vi "Phasor Get Min, Med & Max Decay Indices.vi"(8 "Period":dbl, 9 "Max X":dbl, 10 "Min X":dbl, 11 "X Array":dbl[](array[numeric])) -> (1 "Max X idx":dbl, 2 "Med X idx":dbl, 3 "Min X idx":dbl)   [LabVIEW 2021, in "Phasor.lvlib"]
uses:
  Phasor.lvlib
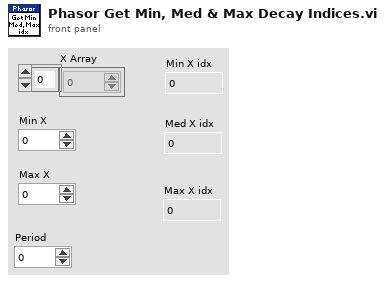
[diagram p1: front panel]
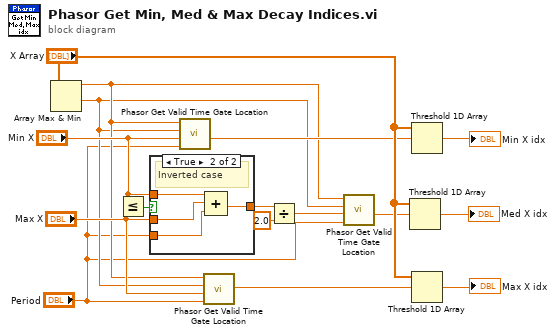
[diagram p0: block diagram]
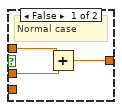
[diagram p2: hidden frame]
diagram:
  n1 = Array Max & Min(array="X Array") -> (max value=w4:dbl, min value=w3:dbl)  [unwired: 2 out]
  n2 = Less Or Equal?(x="Min X", y="Max X") -> (x <= y?=w12:bool)
  n3 = case shown="True" w12 {
    tunnel: "Min X" -> [w19 w23]
    tunnel: "Max X" -> [w18 w22]
    tunnel: "Period" -> [_ w20]
    tunnel: [w17 w21] -> w10
    frame False {
      # "Normal case"
      n4 = Add(x=w19, y=w18) -> (x+y=w17:dbl)
    }
    frame True {
      # "Inverted case"
      n5 = Compound Arithmetic op=ADD(w23, w22, w20) -> (w21:dbl)
    }
  }
  n6 = call "Phasor Get Valid Time Gate Location.vi"("Period"="Period", "X"="Min X", "Min X"=w3, "Max X"=w4) -> ("X in [Min X, Max X]"=w6:dbl)  [unwired: 7 in]
  n7 = call "Phasor Get Valid Time Gate Location.vi"("Period"="Period", "X"="Max X", "Min X"=w3, "Max X"=w4) -> ("X in [Min X, Max X]"=w9:dbl)  [unwired: 7 in]
  n8 = Divide(x=w10, y=2.0) -> (x/y=w5:dbl)
  n9 = call "Phasor Get Valid Time Gate Location.vi"("Period"="Period", "X"=w5, "Min X"=w3, "Max X"=w4) -> ("X in [Min X, Max X]"=w1:dbl)  [unwired: 7 in]
  n10 = Threshold 1D Array(2:w1, 3:"X Array") -> (0:→"Med X idx":dbl)  [unwired: 1 in]
  n11 = Threshold 1D Array(2:w6, 3:"X Array") -> (0:→"Min X idx":dbl)  [unwired: 1 in]
  n12 = Threshold 1D Array(2:w9, 3:"X Array") -> (0:→"Max X idx":dbl)  [unwired: 1 in]
